vi "append_data.vi"(8 "error in (no error)":errorcluster, 10 "archive":T2, 11 "ref in":T1 format="%.0x") -> (0 "error out":errorcluster, 3 "ref out":T1 format="%.0x")   [LabVIEW 2020]
uses:
  archive.ctl
  sync_type_def.ctl
  HT_type-def.ctl
  HF_type_def.ctl
  vacuum_type_def.ctl
  modulator_type_def.ctl
  water_cooling_type_def.ctl
  all_magnets_type_def.ctl
  <vilib>/addons/h5labview2/base/hid_t.ctl
  <vilib>/addons/h5labview2/base/lib_path.vi
  <vilib>/addons/h5labview2/base/H5Equery.vi
  <vilib>/addons/h5labview2/dataset/H5Dread.llb/H5Dread.xnode
  <vilib>/addons/h5labview2/dataset/H5D.lvlib
  <vilib>/addons/h5labview2/group/H5G.lvlib
panel:
  out "error out 2":errorcluster
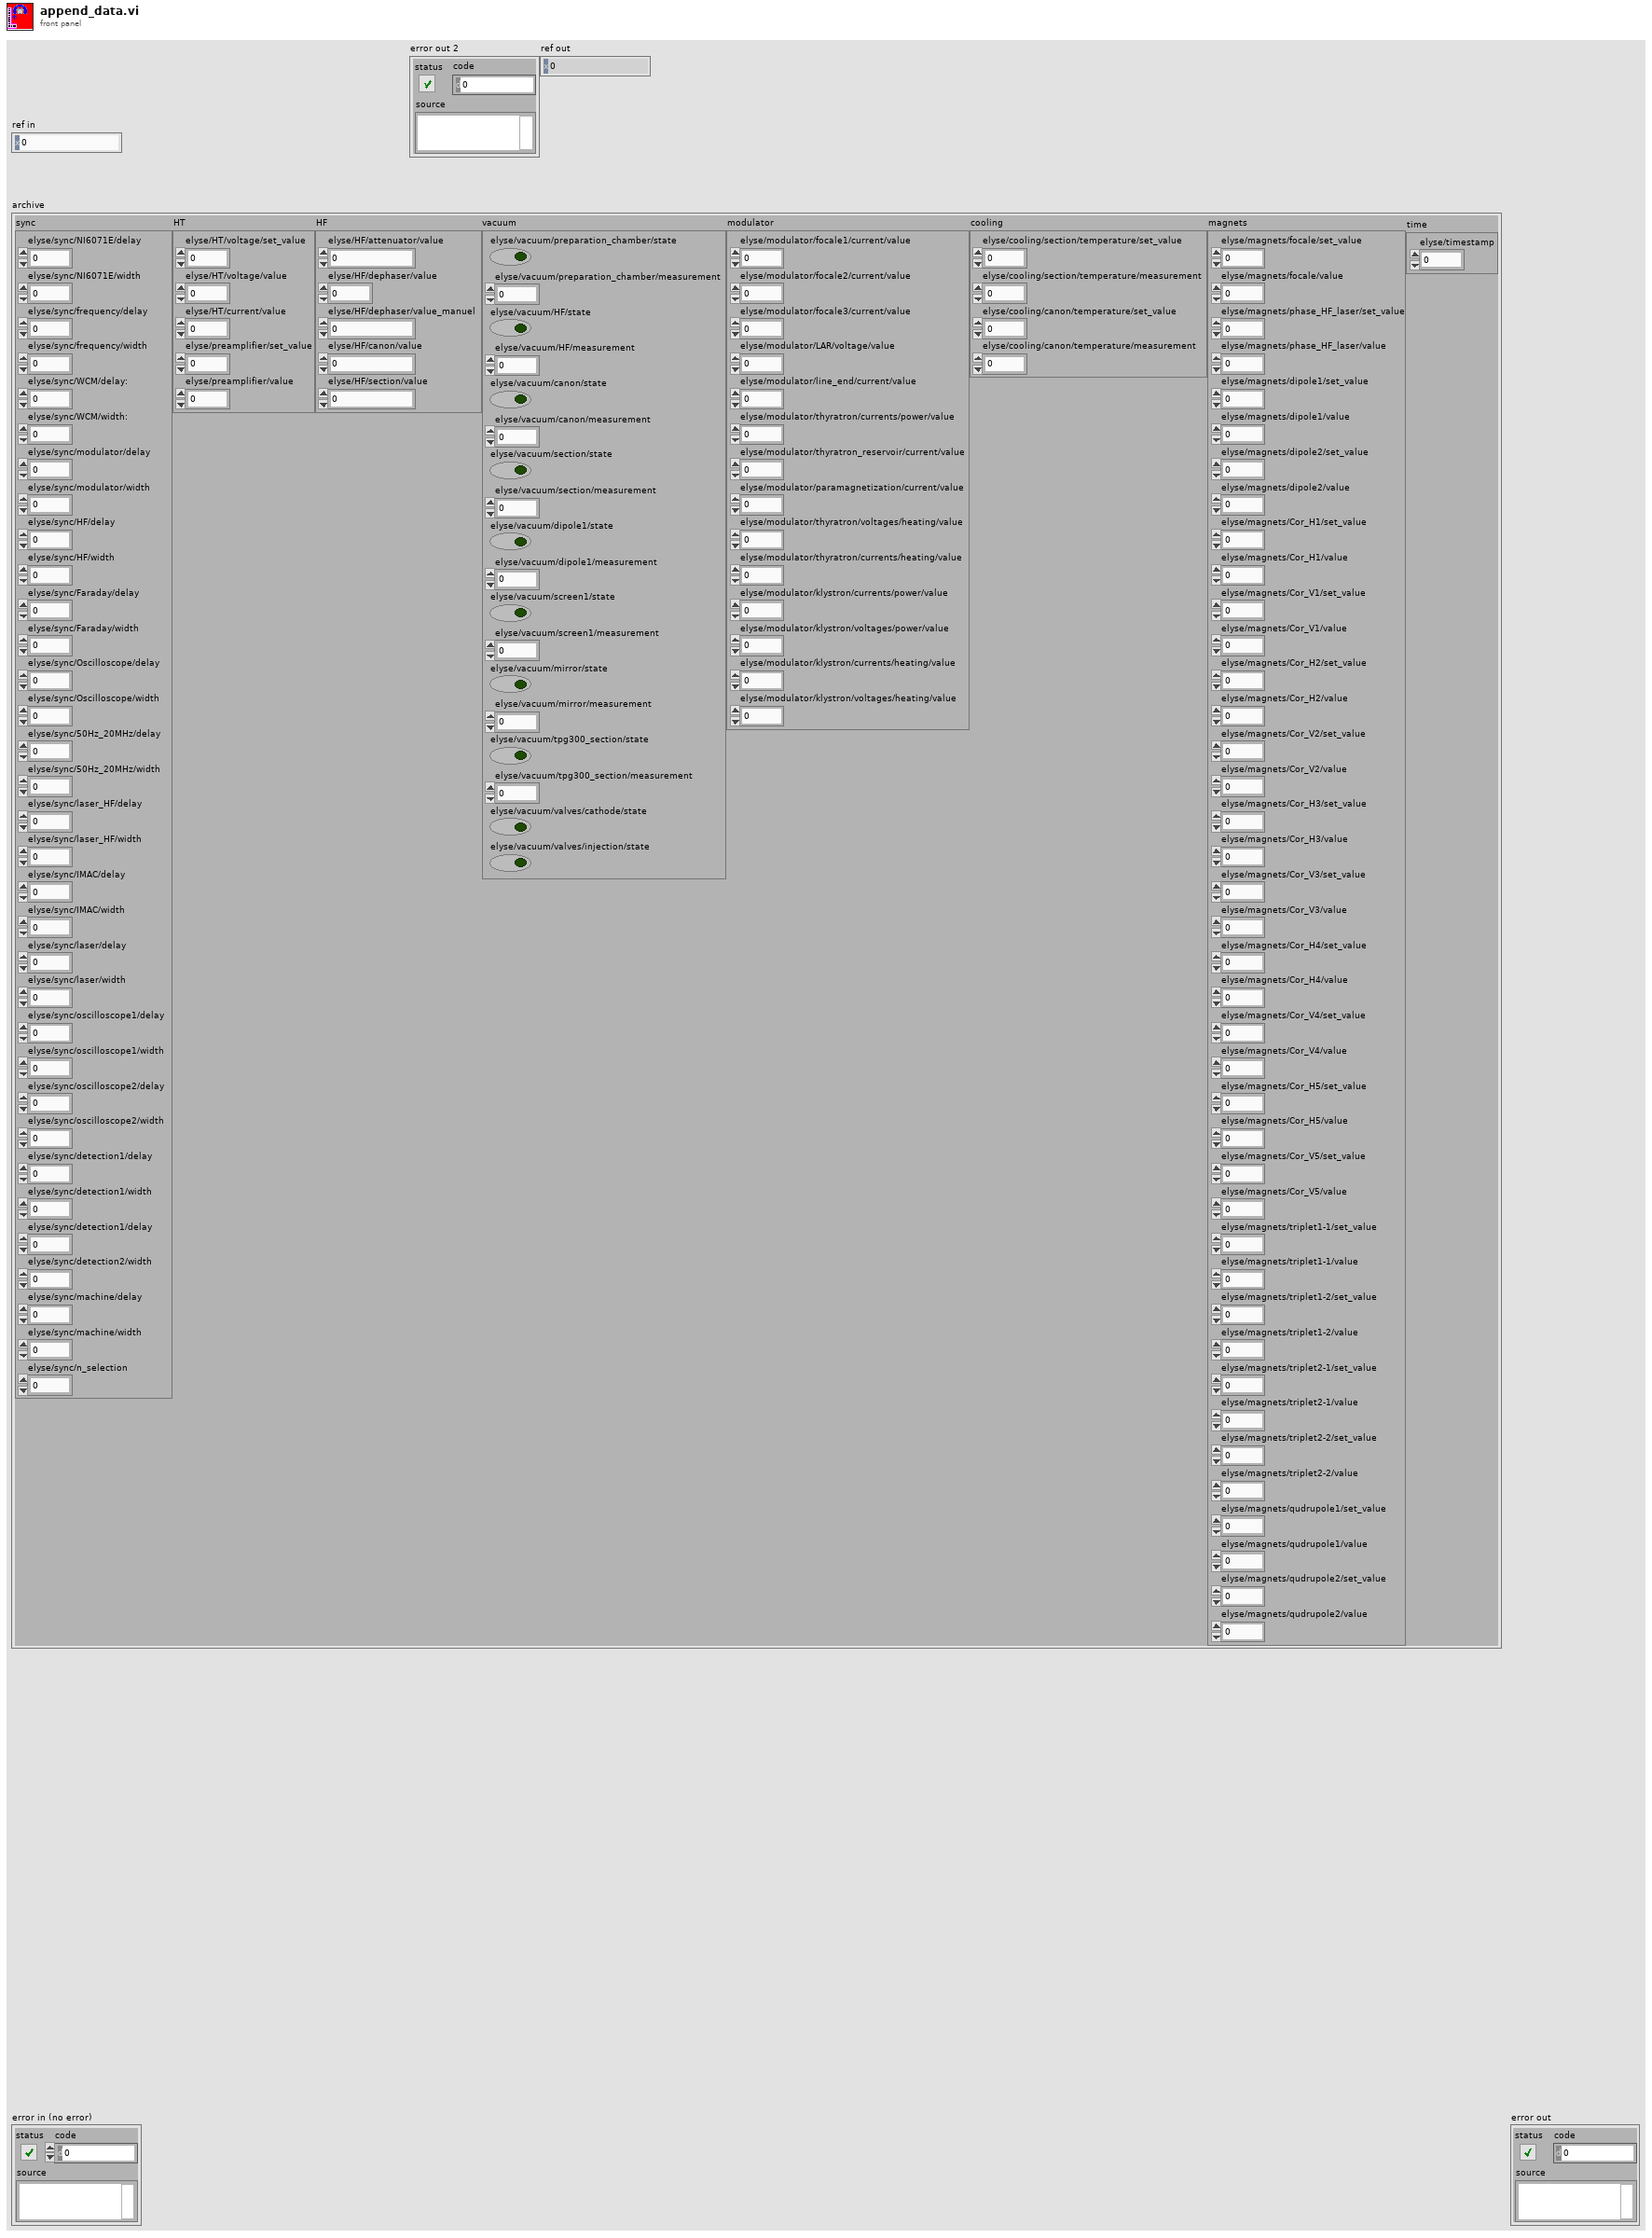
[diagram p1: front panel]
types:
  T1 = typedef "hid_t.ctl" = i64
  T2 = typedef "archive.ctl" = cluster{"sync":T3, "HT":T4, "HF":T5, "vacuum":T6, "modulator":T7, "cooling":T8, "magnets":T9, "time":cluster{"elyse/timestamp":dbl}}
  T3 = typedef "sync_type_def.ctl" = cluster{"elyse/sync/NI6071E/delay":dbl, "elyse/sync/NI6071E/width":dbl, "elyse/sync/frequency/delay":dbl, "elyse/sync/frequency/width":dbl, "elyse/sync/WCM/delay:":dbl, "elyse/sync/WCM/width:":dbl, "elyse/sync/modulator/delay":dbl, "elyse/sync/modulator/width":dbl, "elyse/sync/HF/delay":dbl, "elyse/sync/HF/width":dbl, "elyse/sync/Faraday/delay":dbl, "elyse/sync/Faraday/width":dbl, "elyse/sync/Oscilloscope/delay":dbl, "elyse/sync/Oscilloscope/width":dbl, "elyse/sync/50Hz_20MHz/delay":dbl, "elyse/sync/50Hz_20MHz/width":dbl, "elyse/sync/laser_HF/delay":dbl, "elyse/sync/laser_HF/width":dbl, "elyse/sync/IMAC/delay":dbl, "elyse/sync/IMAC/width":dbl, "elyse/sync/laser/delay":dbl, "elyse/sync/laser/width":dbl, "elyse/sync/oscilloscope1/delay":dbl, "elyse/sync/oscilloscope1/width":dbl, "elyse/sync/oscilloscope2/delay":dbl, "elyse/sync/oscilloscope2/width":dbl, "elyse/sync/detection1/delay":dbl, "elyse/sync/detection1/width":dbl, "elyse/sync/detection1/delay":dbl, "elyse/sync/detection2/width":dbl, "elyse/sync/machine/delay":dbl, "elyse/sync/machine/width":dbl, "elyse/sync/n_selection":dbl}
  T4 = typedef "HT_type-def.ctl" = cluster{"elyse/HT/voltage/set_value":dbl, "elyse/HT/voltage/value":dbl, "elyse/HT/current/value":dbl, "elyse/preamplifier/set_value":dbl, "elyse/preamplifier/value":dbl}
  T5 = typedef "HF_type_def.ctl" = cluster{"elyse/HF/attenuator/value":dbl, "elyse/HF/dephaser/value":dbl, "elyse/HF/dephaser/value_manuel":dbl, "elyse/HF/canon/value":dbl, "elyse/HF/section/value":dbl}
  T6 = typedef "vacuum_type_def.ctl" = cluster{"elyse/vacuum/preparation_chamber/state":bool, "elyse/vacuum/preparation_chamber/measurement":dbl, "elyse/vacuum/HF/state":bool, "elyse/vacuum/HF/measurement":dbl, "elyse/vacuum/canon/state":bool, "elyse/vacuum/canon/measurement":dbl, "elyse/vacuum/section/state":bool, "elyse/vacuum/section/measurement":dbl, "elyse/vacuum/dipole1/state":bool, "elyse/vacuum/dipole1/measurement":dbl, "elyse/vacuum/screen1/state":bool, "elyse/vacuum/screen1/measurement":dbl, "elyse/vacuum/mirror/state":bool, "elyse/vacuum/mirror/measurement":dbl, "elyse/vacuum/tpg300_section/state":bool, "elyse/vacuum/tpg300_section/measurement":dbl, "elyse/vacuum/valves/cathode/state":bool, "elyse/vacuum/valves/injection/state":bool}
  T7 = typedef "modulator_type_def.ctl" = cluster{"elyse/modulator/focale1/current/value":dbl, "elyse/modulator/focale2/current/value":dbl, "elyse/modulator/focale3/current/value":dbl, "elyse/modulator/LAR/voltage/value":dbl, "elyse/modulator/line_end/current/value":dbl, "elyse/modulator/thyratron/currents/power/value":dbl, "elyse/modulator/thyratron_reservoir/current/value":dbl, "elyse/modulator/paramagnetization/current/value":dbl, "elyse/modulator/thyratron/voltages/heating/value":dbl, "elyse/modulator/thyratron/currents/heating/value":dbl, "elyse/modulator/klystron/currents/power/value":dbl, "elyse/modulator/klystron/voltages/power/value":dbl, "elyse/modulator/klystron/currents/heating/value":dbl, "elyse/modulator/klystron/voltages/heating/value":dbl}
  T8 = typedef "water_cooling_type_def.ctl" = cluster{"elyse/cooling/section/temperature/set_value":dbl, "elyse/cooling/section/temperature/measurement":dbl, "elyse/cooling/canon/temperature/set_value":dbl, "elyse/cooling/canon/temperature/measurement":dbl}
  T9 = typedef "all_magnets_type_def.ctl" = cluster{"elyse/magnets/focale/set_value":dbl, "elyse/magnets/focale/value":dbl, "elyse/magnets/phase_HF_laser/set_value":dbl, "elyse/magnets/phase_HF_laser/value":dbl, "elyse/magnets/dipole1/set_value":dbl, "elyse/magnets/dipole1/value":dbl, "elyse/magnets/dipole2/set_value":dbl, "elyse/magnets/dipole2/value":dbl, "elyse/magnets/Cor_H1/set_value":dbl, "elyse/magnets/Cor_H1/value":dbl, "elyse/magnets/Cor_V1/set_value":dbl, "elyse/magnets/Cor_V1/value":dbl, "elyse/magnets/Cor_H2/set_value":dbl, "elyse/magnets/Cor_H2/value":dbl, "elyse/magnets/Cor_V2/set_value":dbl, "elyse/magnets/Cor_V2/value":dbl, "elyse/magnets/Cor_H3/set_value":dbl, "elyse/magnets/Cor_H3/value":dbl, "elyse/magnets/Cor_V3/set_value":dbl, "elyse/magnets/Cor_V3/value":dbl, "elyse/magnets/Cor_H4/set_value":dbl, "elyse/magnets/Cor_H4/value":dbl, "elyse/magnets/Cor_V4/set_value":dbl, "elyse/magnets/Cor_V4/value":dbl, "elyse/magnets/Cor_H5/set_value":dbl, "elyse/magnets/Cor_H5/value":dbl, "elyse/magnets/Cor_V5/set_value":dbl, "elyse/magnets/Cor_V5/value":dbl, "elyse/magnets/triplet1-1/set_value":dbl, "elyse/magnets/triplet1-1/value":dbl, "elyse/magnets/triplet1-2/set_value":dbl, "elyse/magnets/triplet1-2/value":dbl, "elyse/magnets/triplet2-1/set_value":dbl, "elyse/magnets/triplet2-1/value":dbl, "elyse/magnets/triplet2-2/set_value":dbl, "elyse/magnets/triplet2-2/value":dbl, "elyse/magnets/qudrupole1/set_value":dbl, "elyse/magnets/qudrupole1/value":dbl, "elyse/magnets/qudrupole2/set_value":dbl, "elyse/magnets/qudrupole2/value":dbl}
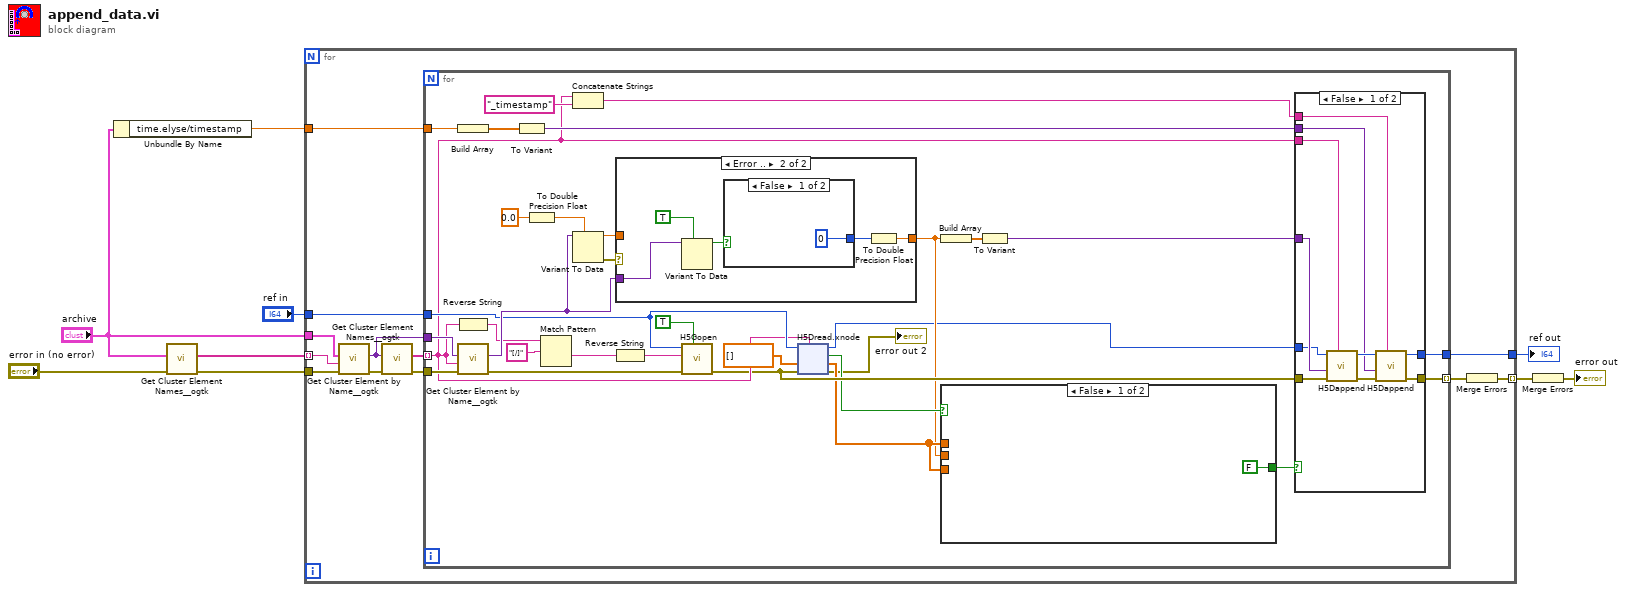
[diagram p0: block diagram]
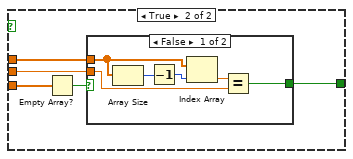
[diagram p3: hidden frame]
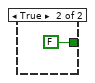
[diagram p4: hidden frame]
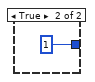
[diagram p6: hidden frame]
diagram:
  n1 = Unbundle By Name("archive") -> ("time.elyse/timestamp"=w2:dbl)
  n2 = call <userlib>:"Get Cluster Element Names__ogtk.vi"("error in (no error)"="error in (no error)", "Cluster"="archive") -> ("error out"=w6:errorcluster, "Element Names"=w8:string[])  [unwired: 8 in]
  n3 = for {
    tunnel: w6 -> [w15]
    tunnel: "ref in" -> [w21]
    tunnel: w8 -> [w18] mode=indexing
    tunnel: "archive" -> [w17]
    tunnel: [w12] -> w5 mode=indexing
    tunnel: w2 -> [w11]
    tunnel: [w10] -> w1
    n4 = call <userlib>:"Get Cluster Element by Name__ogtk.vi"("error in (no error)"=w15, "Element Name"=w18, "Cluster"=w17) -> ("error out"=w14:errorcluster, "VElement"=w16:variant)  [unwired: 6 in, 1 out]
    n5 = call <userlib>:"Get Cluster Element Names__ogtk.vi"("error in (no error)"=w14, "Cluster"=w16) -> ("error out"=w13:errorcluster, "Element Names"=w20:string[])  [unwired: 8 in]
    n6 = for {
      tunnel: w21 -> [w32]
      tunnel: w20 -> [w31] mode=indexing
      tunnel: w16 -> [w53]
      tunnel: [w33] -> w19 mode=indexing
      tunnel: w13 -> [w52]
      tunnel: w11 -> [w35]
      tunnel: [w23] -> w10
      n7 = Build Array(w35) -> (w38:dbl[])
      n8 = Reverse String(1:w31) -> (0:w42:string)
      n9 = call <userlib>:"Get Cluster Element by Name__ogtk.vi"("error in (no error)"=w52, "Element Name"=w31, "Cluster"=w53) -> ("error out"=w43:errorcluster, "VElement"=w48:variant)  [unwired: 6 in, 1 out]
      n10 = To Variant(anything=w38) -> (Variant=w34:variant)
      n11 = To Double Precision Float(number=0.0) -> (double precision float=w50:dbl)
      n12 = Match Pattern(string=w42, regular expression="[/]") -> (after substring=w40:string)  [unwired: 1 in, 3 out]
      n13 = Concatenate Strings(w31, "_timestamp" ("string")) -> (w36:string)
      n14 = Variant To Data(type=w50, Variant=w48) -> (data=w47:dbl, error out=w49:errorcluster)  [unwired: 1 in]
      n15 = Reverse String(1:w40) -> (0:w39:string)
      n16 = case shown="Error .." w49 {
        tunnel: w48 -> [_ w99]
        tunnel: [w94 w95] -> w26
        tunnel: w47 -> [w94 _]
        frame No Error {
        }
        frame Error {
          n17 = Variant To Data(type=TRUE, Variant=w99) -> (data=w97:bool)  [unwired: 1 in, 1 out]
          n18 = case shown="False" w97 {
            tunnel: [0 1] -> w96
            frame False {
            }
            frame True {
            }
          }
          n19 = To Double Precision Float(number=w96) -> (double precision float=w95:dbl)
        }
      }
      n20 = call <vilib>:"H5Gopen.vi"("create? (F)"=TRUE, "error in (no error)"=w43, "name"=w39, "ref in"=w32) -> ("error out"=w29:errorcluster)  [unwired: 6 in, 1 out]
      n21 = xnode "H5Dread.xnode"("dataset name (this)"=w31, "error in (no error)"=w29, "default"=dbl[] [], "ref in"=w32) -> ("error out"=→"error out 2":errorcluster, "data"=w27:dbl[], "found?"=w28:bool, "ref out"=w22:i64)  [unwired: 2 in]
      n22 = Build Array(w26) -> (w46:dbl[])
      n23 = case shown="False" w28 {
        tunnel: w27 -> [_ w70]
        tunnel: w27 -> [_ w69]
        tunnel: w26 -> [_ w68]
        tunnel: [FALSE w67] -> w25
        frame False {
        }
        frame True {
          n24 = Empty Array?(array=w70) -> (empty?=w71:bool)
          n25 = case shown="False" w71 {
            tunnel: w69 -> [w77 _]
            tunnel: w68 -> [w73 _]
            tunnel: [w72 FALSE] -> w67
            frame False {
              n26 = Array Size(array=w77) -> (size(s)=w76:i32)
              n27 = Decrement(x=w76) -> (x-1=w75:i32)
              n28 = Index Array(array=w77, index=w75) -> (element=w74:dbl)
              n29 = Equal?(x=w74, y=w73) -> (x = y?=w72:bool)
            }
            frame True {
            }
          }
        }
      }
      n30 = To Variant(anything=w46) -> (Variant=w45:variant)
      n31 = case shown="False" w25 {
        tunnel: w45 -> [w63 _]
        tunnel: w36 -> [w61 _]
        tunnel: w34 -> [w59 _]
        tunnel: [w58 w65] -> w33
        tunnel: w31 -> [w57 _]
        tunnel: w29 -> [w56 w65]
        tunnel: [w55 w64] -> w23
        tunnel: w22 -> [w54 w64]
        frame False {
          n32 = call <vilib>:"H5Dappend.vi"("dataset name"=w57, "error in (no error)"=w56, "data"=w63, "ref in"=w54) -> ("error out"=w62:errorcluster, "ref out"=w60:T1)  [unwired: 4 in, 2 out]
          n33 = call <vilib>:"H5Dappend.vi"("dataset name"=w61, "error in (no error)"=w62, "data"=w59, "ref in"=w60) -> ("error out"=w58:errorcluster, "ref out"=w55:T1)  [unwired: 4 in, 2 out]
        }
        frame True {
        }
      }
    }
    n34 = Merge Errors(w19) -> (w12:errorcluster)
  }
  "ref out" <- w1
  n35 = Merge Errors(w5) -> (→"error out":errorcluster)
